vi "Workspace Update UI Objects.vi"(8 "error in (no error)":errorcluster, 10 "Values":dbl[](array[numeric]), 11 "UI.Refs":T1) -> (0 "error out":errorcluster)   [LabVIEW 2015, in "Diagnostics Addon Shared.lvlib"]
uses:
  Types/UI.Refs.ctl
  Types/Channel Commands Enum.ctl
  Diagnostics Addon Shared.lvlib
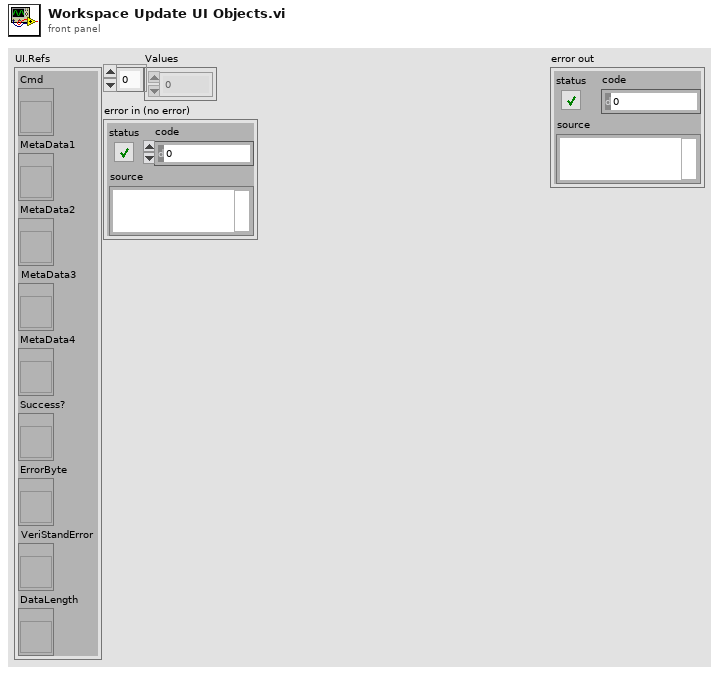
[diagram p1: front panel]
types:
  T1 = typedef "Diagnostics Addon Shared.lvlib/UI.Refs.ctl" = cluster{"Cmd":refnum<vi>, "MetaData1":refnum<vi>, "MetaData2":refnum<vi>, "MetaData3":refnum<vi>, "MetaData4":refnum<vi>, "Success?":refnum<vi>, "ErrorByte":refnum<vi>, "VeriStandError":refnum<vi>, "DataLength":refnum<vi>}
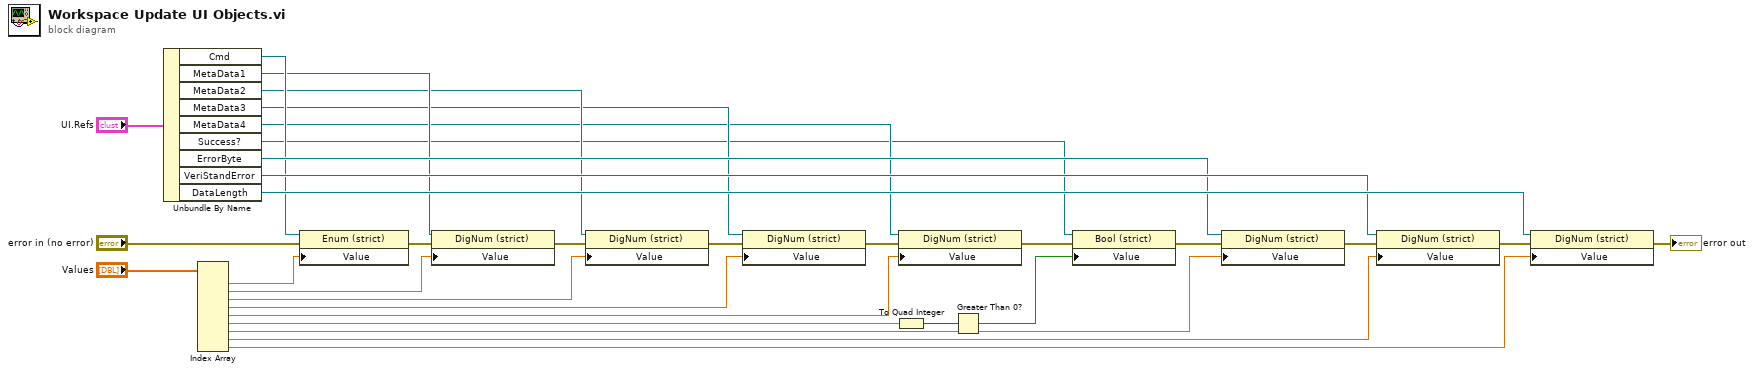
[diagram p0: block diagram]
diagram:
  n1 = Unbundle By Name("UI.Refs") -> ("Cmd"=w26:refnum<vi>, "MetaData1"=w25:refnum<vi>, "MetaData2"=w24:refnum<vi>, "MetaData3"=w23:refnum<vi>, "MetaData4"=w19:refnum<vi>, "Success?"=w17:refnum<vi>, "ErrorByte"=w28:refnum<vi>, "VeriStandError"=w30:refnum<vi>, "DataLength"=w31:refnum<vi>)
  n2 = Index Array(array="Values") -> (element #1=w11:dbl, element #2=w10:dbl, element #3=w9:dbl, element #4=w8:dbl, element #5=w7:dbl, element #6=w6:dbl, element #7=w3:dbl, element #8=w2:dbl, element #9=w1:dbl)  [unwired: 9 in]
  n3 = property class="Enum (strict)"(reference=w26, error in="error in (no error)", "Value"=w11) -> (error out=w22:errorcluster)  [unwired: 1 out]
  n4 = property class="DigNum (strict)"(reference=w25, error in=w22, "Value"=w10) -> (error out=w21:errorcluster)  [unwired: 1 out]
  n5 = property class="DigNum (strict)"(reference=w24, error in=w21, "Value"=w9) -> (error out=w20:errorcluster)  [unwired: 1 out]
  n6 = property class="DigNum (strict)"(reference=w23, error in=w20, "Value"=w8) -> (error out=w18:errorcluster)  [unwired: 1 out]
  n7 = To Quad Integer(1:w6) -> (0:w4:i64)
  n8 = property class="DigNum (strict)"(reference=w19, error in=w18, "Value"=w7) -> (error out=w16:errorcluster)  [unwired: 1 out]
  n9 = Greater Than 0?(x=w4) -> (x > 0?=w5:bool)
  n10 = property class="Bool (strict)"(reference=w17, error in=w16, "Value"=w5) -> (error out=w15:errorcluster)  [unwired: 1 out]
  n11 = property class="DigNum (strict)"(reference=w28, error in=w15, "Value"=w3) -> (error out=w27:errorcluster)  [unwired: 1 out]
  n12 = property class="DigNum (strict)"(reference=w30, error in=w27, "Value"=w2) -> (error out=w29:errorcluster)  [unwired: 1 out]
  n13 = property class="DigNum (strict)"(reference=w31, error in=w29, "Value"=w1) -> (error out=→"error out":errorcluster)  [unwired: 1 out]
